vi "Read MFC.vi"(8 "error in (no error)":errorcluster, 11 "MFC in":refnum<class "MFC.lvclass">) -> (0 "error out":errorcluster, 3 "MFC out":refnum<class "MFC.lvclass">)   [LabVIEW 2013, in "MFC.LVLIB" / "MFC.lvclass"]
uses:
  MFC.lvclass
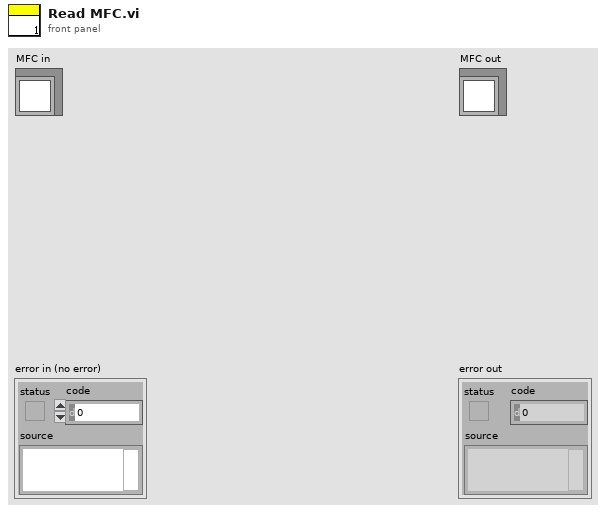
[diagram p1: front panel]
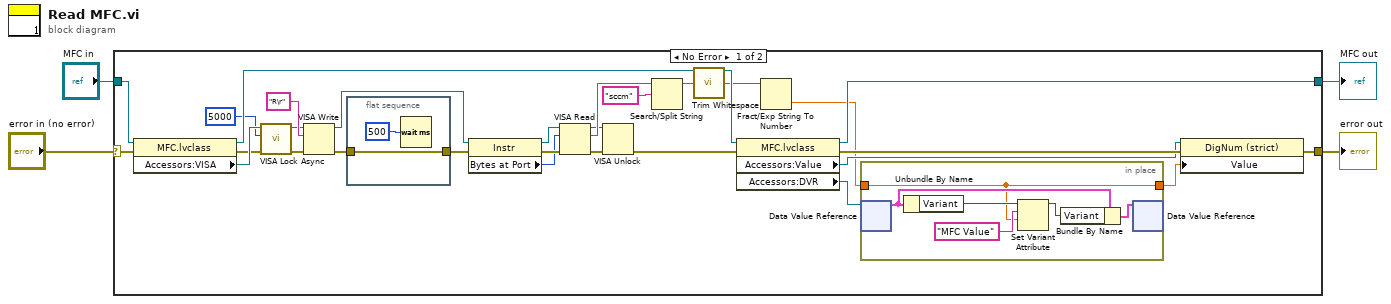
[diagram p0: block diagram]
diagram:
  n1 = case shown="No Error" "error in (no error)" {
    selector: "error in (no error)" -> [w32 w43]
    tunnel: [w5 w43] -> w3
    tunnel: [w29 w42] -> w1
    tunnel: "MFC in" -> [w33 w42]
    frame No Error {
      n2 = property class="MFC.lvclass"(reference=w33, error in=w32) -> (reference out=w30:refnum<class "MFC.lvclass">, error out=w10:errorcluster, "Accessors:VISA"=w13:refnum<visa-resource-name>)
      n3 = call <vilib>:"VISA Lock Async.vi"("error in (no error)"=w10, "timeout (0)"=u32 5000, "VISA resource name"=w13) -> ("error out"=w11:errorcluster, "VISA resource name out"=w12:refnum<visa-resource-name>)  [unwired: 6 in, 1 out]
      n4 = VISA Write(VISA resource name=w12, write buffer="R\r", error in (no error)=w11) -> (VISA resource name out=w27:refnum<visa-resource-name>, error out=w24:errorcluster)  [unwired: 1 out]
      n5 = flat-sequence {
        tunnel: [w40] -> w25
        tunnel: w24 -> [w40]
        frame #0 {
          n6 = Wait (ms)(milliseconds to wait=u32 500) -> ()  [unwired: 1 out]
        }
      }
      n7 = property class="Instr"(reference=w27, error in=w25) -> (reference out=w28:refnum<visa-resource-name>, error out=w26:errorcluster, "Bytes at Port"=w22:u32)
      n8 = VISA Read(VISA resource name=w28, byte count=w22, error in (no error)=w26) -> (VISA resource name out=w8:refnum<visa-resource-name>, read buffer=w18:string, error out=w7:errorcluster)  [unwired: 1 out]
      n9 = VISA Unlock(8:w7, 11:w8) -> (0:w6:errorcluster)  [unwired: 1 out]
      n10 = Search/Split String(string=w18, search string/char (-)="sccm") -> (substring before match=w20:string)  [unwired: 1 in, 2 out]
      n11 = call <vilib>:"Trim Whitespace.vi"("string"=w20) -> ("trimmed string"=w19:string)  [unwired: 1 in]
      n12 = property class="MFC.lvclass"(reference=w30, error in=w6) -> (reference out=w29:refnum<class "MFC.lvclass">, error out=w31:errorcluster, "Accessors:Value"=w16:refnum<vi>, "Accessors:DVR"=w17:refnum<data-value>)
      n13 = Fract/Exp String To Number(string=w19) -> (number=w15:dbl)  [unwired: 3 in, 1 out]
      n14 = in-place {
        in-place-border: w15 -> [w34]
        in-place-border: [w34] -> w14
        n15 = in-place-dvr #1(w17) -> (w36:cluster{"Array":string[], "Variant":variant})  [unwired: 1 out]
        n16 = Unbundle By Name(w36) -> ("Variant"=w38:variant)
        n17 = Set Variant Attribute(Variant=w38, name="MFC Value", value=w34) -> (Variant out=w37:variant)  [unwired: 1 in, 2 out]
        n18 = Bundle By Name(cluster=w36, "Variant"=w37) -> (w39:cluster{"Array":string[], "Variant":variant})
        n19 = in-place-dvr #1(w39) -> ()  [unwired: 2 out]
      }
      n20 = property class="DigNum (strict)"(reference=w16, error in=w31, "Value"=w14) -> (error out=w5:errorcluster)  [unwired: 1 out]
    }
    frame Error {
    }
  }
  "error out" <- w3
  "MFC out" <- w1
